vi "Max & Min.vi"() -> ()   [LabVIEW 2016]
panel:
  out "Min":dbl
  out "Max":dbl
  in  "Y":dbl
  in  "X":dbl
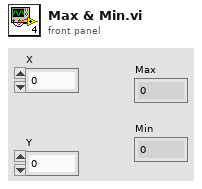
[diagram p1: front panel]
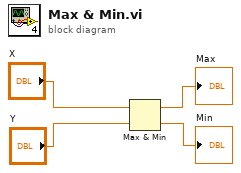
[diagram p0: block diagram]
diagram:
  n1 = Max & Min(x="X", y="Y") -> (max(x,y)=→"Max":dbl, min(x,y)=→"Min":dbl)
